vi "transformation_matrix_to_2D_orthogonal_matrix.vi"(1 "A x B":T1) -> (0 "Real Matrix":T1)   [LabVIEW 2010]
uses:
  <vilib>/Analysis/Matrix/Datatypes/RealMatrix.ctl
  <vilib>/Analysis/7linalg.llb/Create Special Real Matrix.vi
  <vilib>/Analysis/7linalg.llb/Real SVD Decomposition.vi
  <vilib>/Analysis/baseanly.llb/Real A x B.vi
  <vilib>/Analysis/NI_AALPro.lvlib
  <vilib>/Analysis/NI_AALBase.lvlib
  <vilib>/Analysis/Matrix/NI_Matrix.lvlib
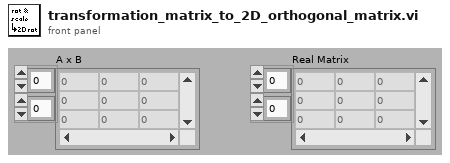
[diagram p1: front panel]
types:
  T1 = typedef "NI_Matrix.lvlib/RealMatrix.ctl" = dbl[][]
  T2 = enum32{"Identity", "Diagonal", "Toepliz", "Vandermonde", "Companion"}
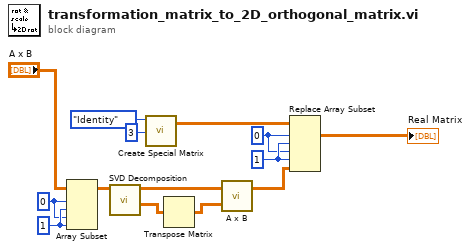
[diagram p0: block diagram]
diagram:
  w13 = 1 ("column N")
  w12 = 0 ("row 1")
  w7 = 1 ("column N")
  w6 = 0 ("row 1")
  n1 = Array Subset(array="A x B", index (row)=w6, length (row)=w7, index (col)=w6, length (col)=w7) -> (w5:T1)
  n2 = call-poly <vilib>:"SVD Decomposition.vi"("A"=w5) -> ("Matrix V"=w2:T1, "Matrix U"=w4:T1)  [unwired: 6 in, 3 out]
  n3 = call-poly <vilib>:"Create Special Matrix.vi"("matrix type"=T2."Identity", "matrix size"=3) -> ("Special Matrix"=w10:T1)  [unwired: 3 in, 1 out]
  n4 = Transpose Matrix(1:w2) -> (0:w3:T1)
  n5 = call-poly <vilib>:"A x B.vi"("B"=w3, "A"=w4) -> ("A x B"=w11:T1)  [unwired: 1 out]
  n6 = Replace Array Subset(array=w10, new element=w11, index (dim 0)=w12, index (dim 1)=w13, index (dim 2)=w12, index (dim 3)=w13) -> (→"Real Matrix":T1)
